vi "PhaseDiff.vi"(4 "angle units":T1 items=["radian in, radian out", "radian in, degree out", "degree in, degree out", "degree in, radian out"], 7 "Angle 2":dbl[](array[numeric]), 8 "Angle 1":dbl[](array[numeric])) -> (3 "Absolute Angle Difference":dbl[](array[numeric]))   [LabVIEW 2013]
uses:
  <vilib>/Analysis/coordinate.llb/Angle Units.ctl
  <vilib>/Analysis/coordinate.llb/Angle Range (Degree).ctl
  <vilib>/Analysis/NI_AAL_Angle.lvlib
panel:
  out "error":i32
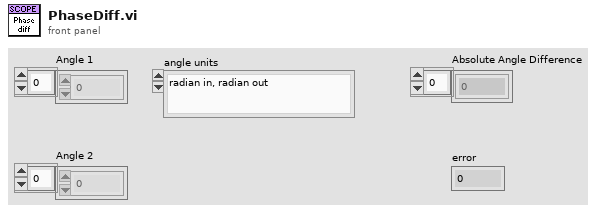
[diagram p1: front panel]
types:
  T1 = typedef "NI_AAL_Angle.lvlib/Angle Units.ctl" = i32
  T2 = typedef "NI_AAL_Angle.lvlib/Angle Range (Degree).ctl" = u16
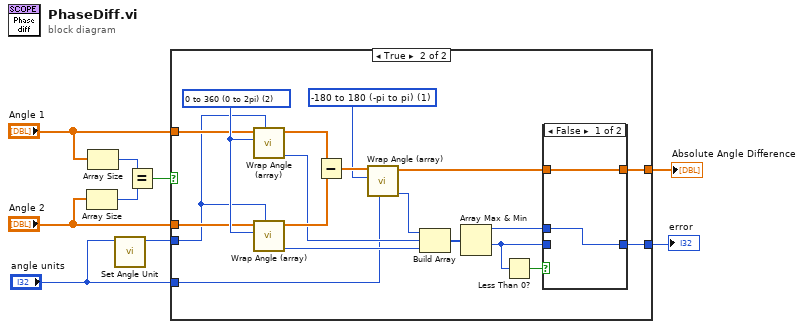
[diagram p0: block diagram]
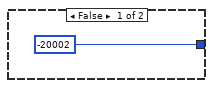
[diagram p2: hidden frame]
diagram:
  n1 = Array Size(array="Angle 2") -> (size(s)=w5:i32)
  n2 = Array Size(array="Angle 1") -> (size(s)=w4:i32)
  n3 = call <vilib>:"Set Angle Unit.vi"("angle units in"="angle units") -> ("angle units out"=w2:T1)  [unwired: 10 in]
  n4 = Equal?(x=w4, y=w5) -> (x = y?=w3:bool)
  n5 = case shown="True" w3 {
    tunnel: [-20002 w18] -> w9
    tunnel: [_ w17] -> w8
    tunnel: "Angle 1" -> [_ w16]
    tunnel: "Angle 2" -> [_ w15]
    tunnel: w2 -> [_ w12]
    tunnel: "angle units" -> [_ w13]
    frame False {
    }
    frame True {
      w14 = T2 1 items=["none", "-180 to 180 (-pi to pi)", "0 to 360 (0 to 2pi)"] ("angle range")
      w29 = T2 2 items=["none", "-180 to 180 (-pi to pi)", "0 to 360 (0 to 2pi)"] ("angle range")
      n6 = call <vilib>:"Wrap Angle (array).vi"("angle units"=w12, "angle range"=w29, "Angle In"=w16) -> ("error"=w25:i32, "Angle Out"=w28:dbl[])  [unwired: 7 in]
      n7 = call <vilib>:"Wrap Angle (array).vi"("angle units"=w12, "angle range"=w29, "Angle In"=w15) -> ("error"=w24:i32, "Angle Out"=w27:dbl[])  [unwired: 7 in]
      n8 = Subtract(x=w28, y=w27) -> (x-y=w26:dbl[])
      n9 = call <vilib>:"Wrap Angle (array).vi"("angle units"=w13, "angle range"=w14, "Angle In"=w26) -> ("error"=w23:i32, "Angle Out"=w11:dbl[])  [unwired: 7 in]
      n10 = Build Array(w23, w25, w24) -> (w22:i32[])
      n11 = Array Max & Min(array=w22) -> (max value=w19:i32, min value=w20:i32)  [unwired: 2 out]
      n12 = Less Than 0?(x=w20) -> (x < 0?=w21:bool)
      n13 = case shown="False" w21 {
        tunnel: w11 -> [w31 _]
        tunnel: [w31 _] -> w17
        tunnel: w20 -> [_ w32]
        tunnel: [w30 w32] -> w18
        tunnel: w19 -> [w30 _]
        frame False {
        }
        frame True {
        }
      }
    }
  }
  "Absolute Angle Difference" <- w8
  "error" <- w9
